vi "solution.vi"() -> ()   [LabVIEW 2015]
doc: "Use this template to build a producer/consumer design pattern with events to produce queue items. Use this design pattern instead of the User Interface Event Handler pattern for user interfaces when you want to execute code asynchronously in response to an event without slowing the user interface responsiveness."
uses:
  Controls/order&data.ctl
  Controls/#status.ctl
  Users Data.ctl
  Controls/User data.ctl
  Controls/Buttons.ctl
  Controls/#status message.ctl
panel:
  in  "error in":errorcluster
  out "error out":errorcluster
  in  "Enter":bool
  in  "User Input":string
  in  "Right Buttons":T1
  out "Right Menu":T2
  in  "Left Buttons":T1
  out "Left Menu":T2
  in  "Card Simulator":bool
  out "ATM Messages":string
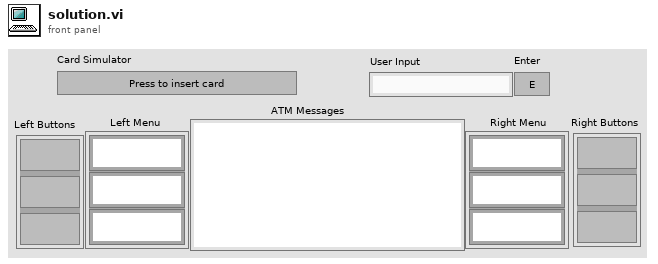
[diagram p1: front panel]
types:
  T1 = cluster{"Func Button":bool, "Func Button 2":bool, "Func Button 3":bool}
  T2 = cluster{"RFS String":string, "RFS String 2":string, "RFS String 3":string}
  T3 = typedef "Buttons.ctl" = cluster{"Left Buttons":cluster{"Func Button":bool, "Func Button 2":bool, "Func Button 3":bool}, "Right Buttons":cluster{"Func Button":bool, "Func Button 2":bool, "Func Button 3":bool}}
  T4 = typedef "Users Data.ctl" = cluster{"Users":T5[], "Customer":T5, "Message":string, "Right Menu":cluster{"RFS String":string, "RFS String 2":string, "RFS String 3":string}, "Left Menu":cluster{"RFS String":string, "RFS String 2":string, "RFS String 3":string}}
  T5 = typedef "User data.ctl" = cluster{"Name":string, "Surname":string, "Cash":i32, "PIN":string}
  T6 = typedef "order&data.ctl" = cluster{"order":T7, "data":string}
  T7 = typedef "#status.ctl" = enum16{"Balance inq", "End of Time", "Show messsage", "Check PIN", "Initialize", "Exit", "Return&Terminate", "Balance Inquiry", "None", "Fast Cash", "Withdraw", "Deposit"}
  T8 = typedef "#status message.ctl" = enum16{"Balance inq", "Withdraw welcome", "Withdraw Failed", "Deposit welcome", "End of Time", "Show messsage", "Check PIN", "Initialize", "Exit", "Return&Terminate", "Balance Inquiry", "None", "First Cash", "Withdraw", "Deposit"}
  T9 = enum8{"Enabled", "Disabled", "Disabled and Grayed Out"}
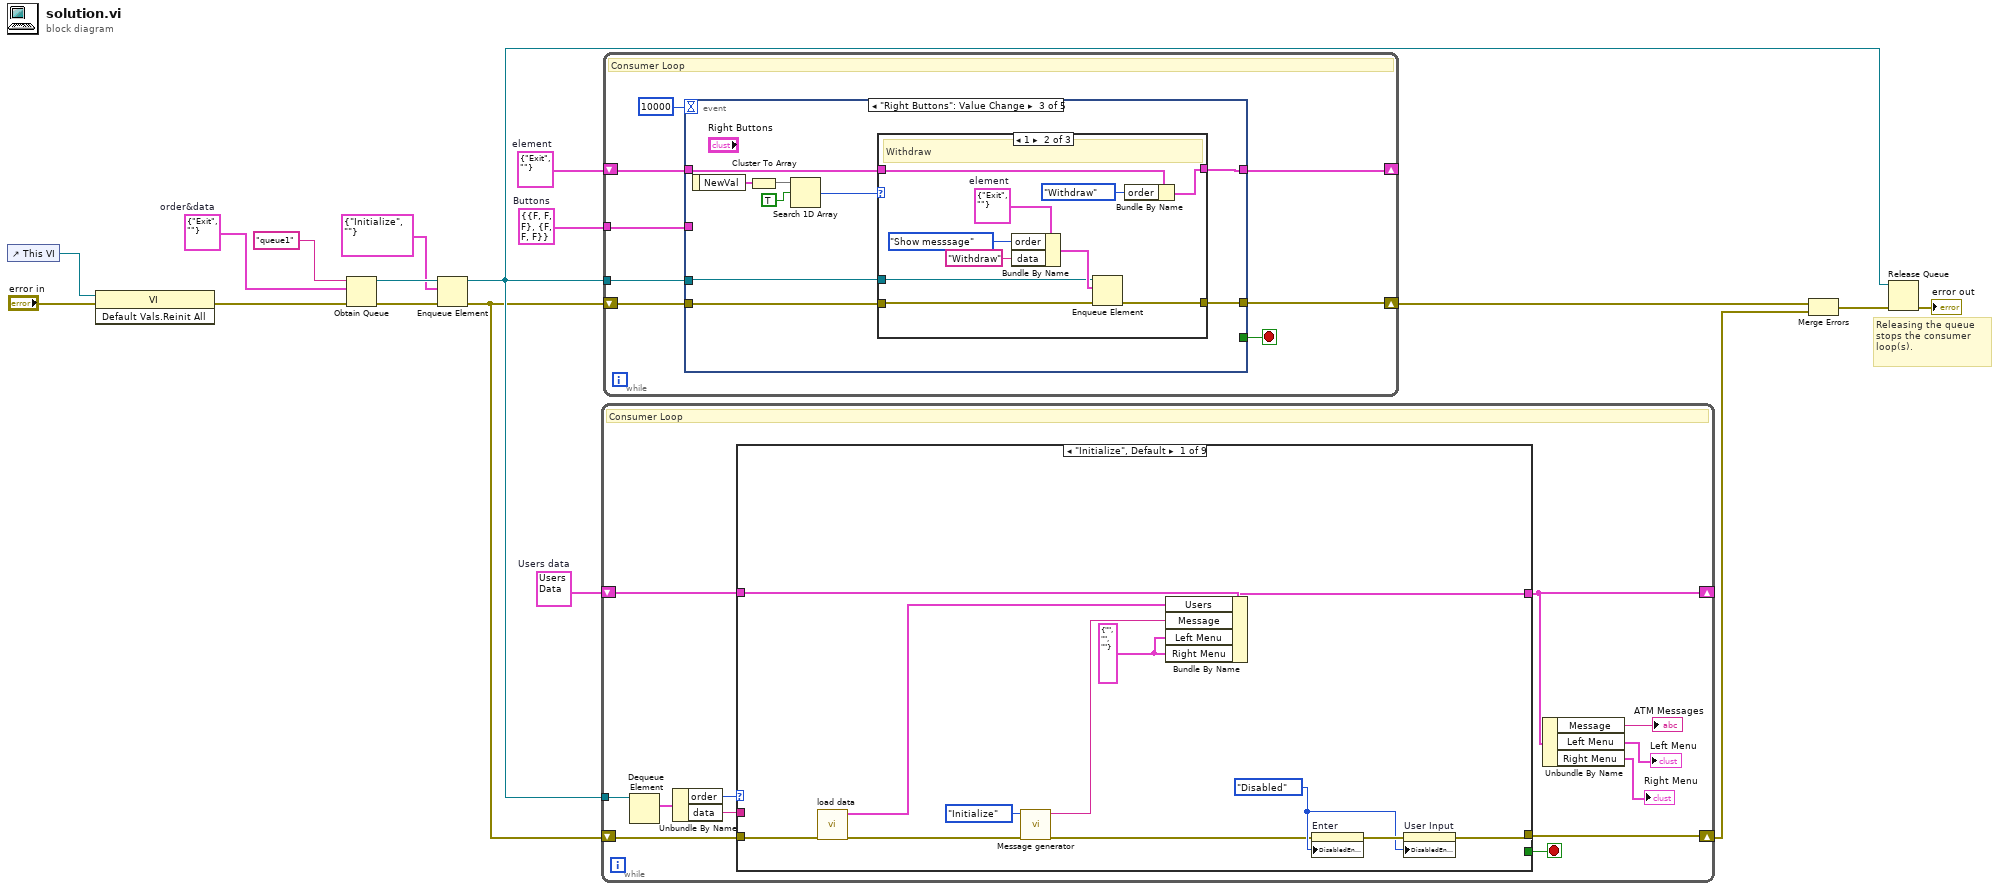
[diagram p0: block diagram]
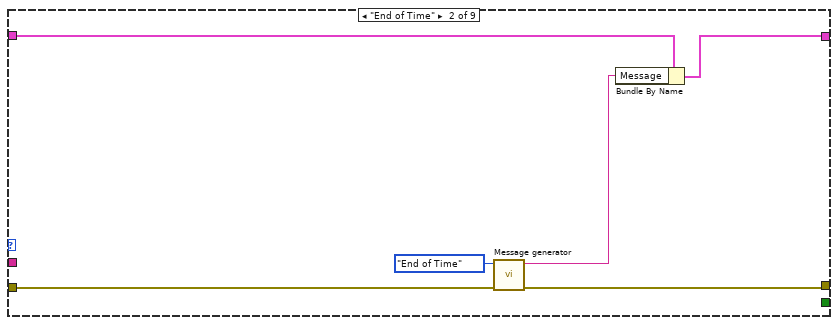
[diagram p2: hidden frame]
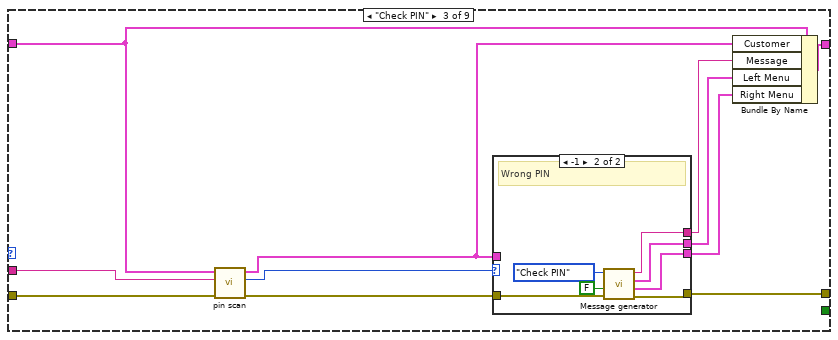
[diagram p3: hidden frame]
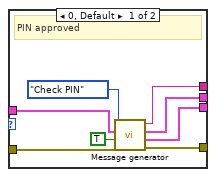
[diagram p4: hidden frame]
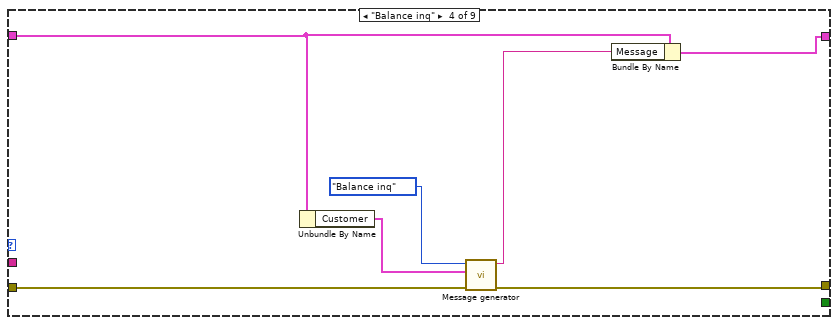
[diagram p5: hidden frame]
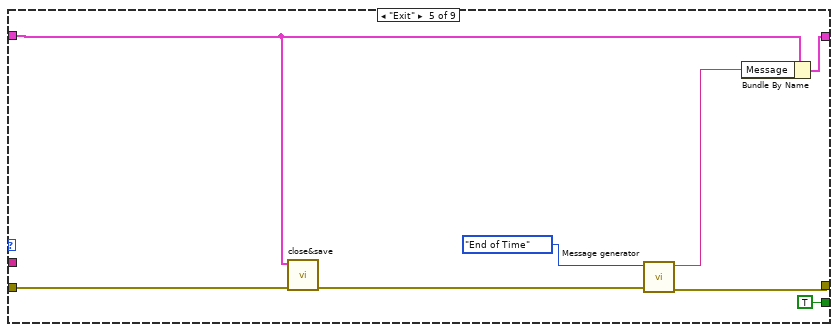
[diagram p6: hidden frame]
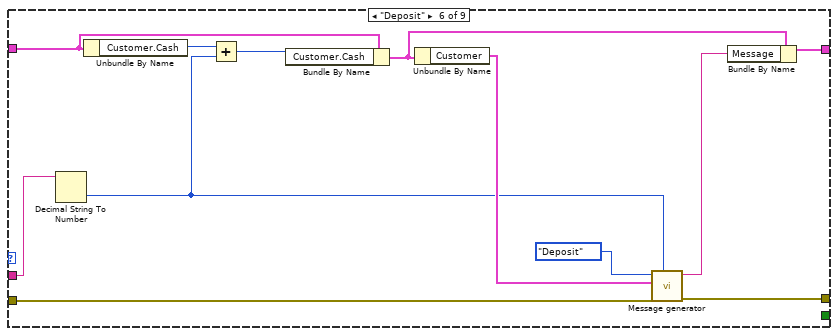
[diagram p7: hidden frame]
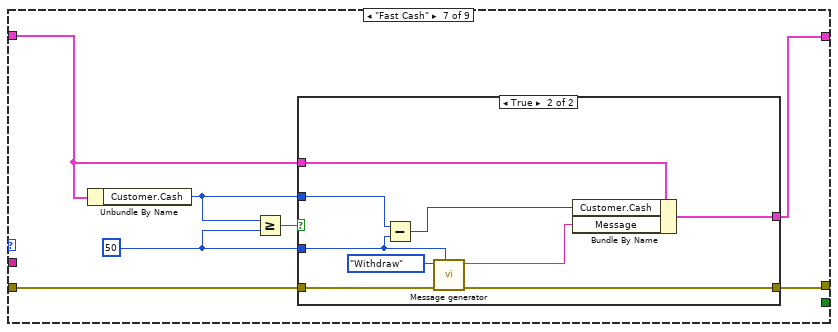
[diagram p8: hidden frame]
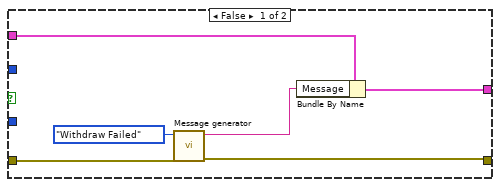
[diagram p9: hidden frame]
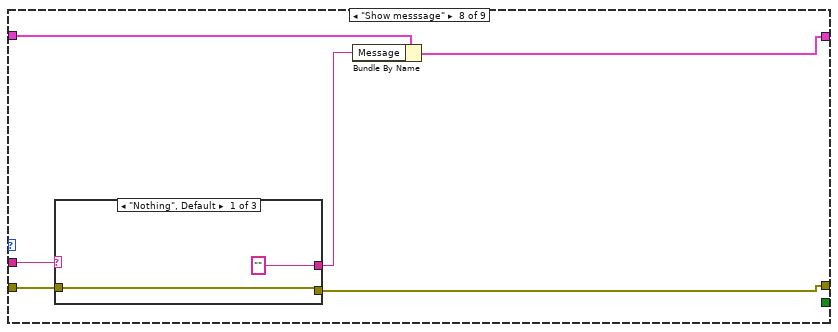
[diagram p10: hidden frame]
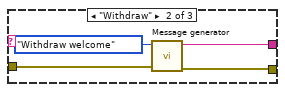
[diagram p11: hidden frame]
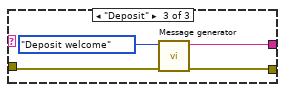
[diagram p12: hidden frame]
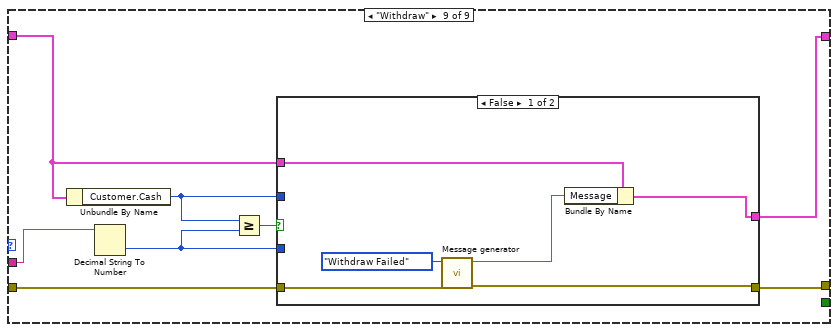
[diagram p13: hidden frame]
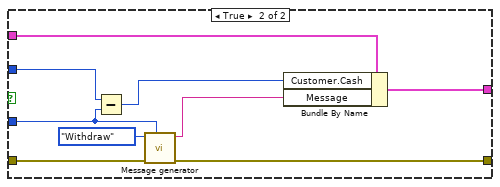
[diagram p14: hidden frame]
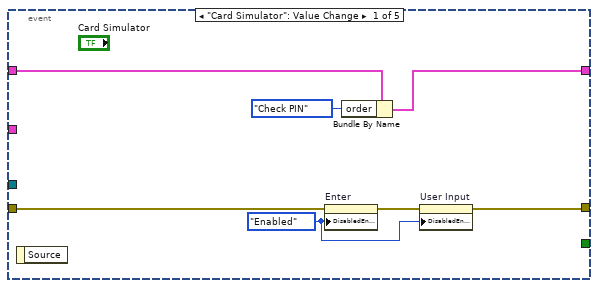
[diagram p15: hidden frame]
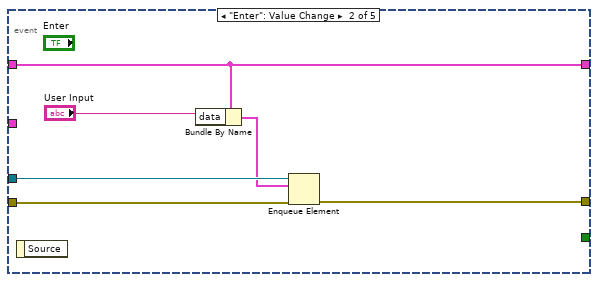
[diagram p16: hidden frame]
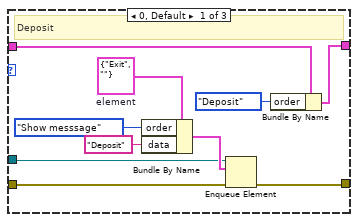
[diagram p17: hidden frame]
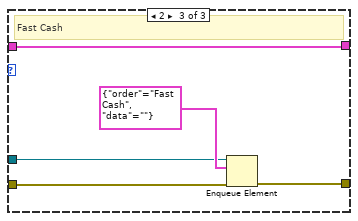
[diagram p18: hidden frame]
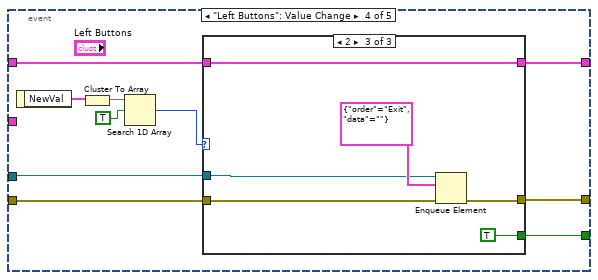
[diagram p19: hidden frame]
diagram:
  w8 = T3 {"Left Buttons"={"Func Button"=FALSE, "Func Button 2"=FALSE, "Func Button 3"=FALSE}, "Right Buttons"={"Func Button"=FALSE, "Func Button 2"=FALSE, "Func Button 3"=FALSE}}  # Buttons
  w9 = T4 {"Users"=[{"Name"="John", "Surname"="Doe", "Cash"=2000, "PIN"=""}, {"Name"="Jennifer", "Surname"="Rodriguez", "Cash"=1500, "PIN"=""}, {"Name"="Bryan", "Surname"="Smith", "Cash"=800, "PIN"=""}, {"Name"="Julie", "Surname"="Ramirez", "Cash"=900, "PIN"=""}], "Customer"={"Name"="", "Surname"="", "Cash"=0, "PIN"=""}, "Message"="", "Right Menu"={"RFS String"="", "RFS String 2"="", "RFS String 3"=""}, "Left Menu"={"RFS String"="", "RFS String 2"="", "RFS String 3"=""}}  # Users data
  w10 = T6 {"order"=enum."Exit", "data"=""}  # element
  w17 = T6 {"order"=enum."Exit", "data"=""}  # order&data
  # "Releasing the queue stops the consumer loop(s)."
  n1 = control-ref of="This VI"() -> (w3:refnum<vi>)
  n2 = invoke class="VI" method="Default Vals.Reinit All"(reference=w3, error in="error in") -> (error out=w2:errorcluster)  [unwired: 1 in, 2 out]
  n3 = Obtain Queue(name (unnamed)="queue1", element data type=w17, error in (no error)=w2) -> (queue out=w14:refnum<queue>, error out=w15:errorcluster)  [unwired: 2 in, 1 out]
  n4 = Enqueue Element(queue=w14, element=T6 {"order"=enum."Initialize", "data"=""} ("order&data 2"), error in (no error)=w15) -> (queue out=w13:refnum<queue>, error out=w11:errorcluster)  [unwired: 1 in, 1 out]
  n5 = while {
    tunnel: w13 -> [w25]
    shift-right: [w22] -> w6
    shift-left: w11 -> [w23]
    shift-right: [w21] -> _
    shift-left: w9 -> [w27]
    stop <- w26 stop-if-true
    # "Consumer Loop"
    n6 = Dequeue Element(queue=w25) -> (element=w29:T6)  [unwired: 2 in, 3 out]
    n7 = Unbundle By Name(w29) -> ("order"=w28:T7, "data"=w24:string)
    n8 = case shown="\"Initialize\", Default" w28 {
      tunnel: w27 -> [w41 w45 w57 w77 w81 w93 w103 w128 w140]
      tunnel: [w39 w44 w55 w75 w87 w95 w102 w127 w139] -> w21
      tunnel: [_ _ _ _ TRUE _ _ _ _] -> w26
      tunnel: w24 -> [_ _ w58 _ _ w100 _ w124 w144]
      tunnel: w23 -> [w34 w47 w49 w80 w83 w97 w105 w126 w146]
      tunnel: [w33 w46 w54 w79 w88 w96 w104 w125 w145] -> w22
      frame "Initialize", Default {
        w31 = T2 {"RFS String"="", "RFS String 2"="", "RFS String 3"=""} ("Left Menu")
        w37 = T9."Disabled" ("Disabled")
        n9 = call "load data.vi"("error in"=w34) -> ("error out"=w36:errorcluster, "Array"=w40:T5[])  [unwired: 9 in]
        n10 = call "Message generator.vi"("error in"=w36, "order"=#status_message."Initialize") -> ("error out"=w35:errorcluster, "message"=w32:string)  [unwired: 6 in, 2 out]
        n11 = Bundle By Name(cluster=w41, "Users"=w40, "Message"=w32, "Left Menu"=w31, "Right Menu"=w31) -> (w39:T4)
        n12 = property on="Enter" class="Bool"(error in=w35, "DisabledEnum"=w37) -> (error out=w38:errorcluster)  [unwired: 1 in, 1 out]
        n13 = property on="User Input" class="Str"(error in=w38, "DisabledEnum"=w37) -> (error out=w33:errorcluster)  [unwired: 1 in, 1 out]
      }
      frame "End of Time" {
        n14 = call "Message generator.vi"("error in"=w47, "order"=#status_message."End of Time") -> ("error out"=w46:errorcluster, "message"=w43:string)  [unwired: 6 in, 2 out]
        n15 = Bundle By Name(cluster=w45, "Message"=w43) -> (w44:T4)
      }
      frame "Check PIN" {
        n16 = call "pin scan.vi"("error in"=w49, "data"=w58, "Users data"=w57) -> ("error out"=w48:errorcluster, "index of element"=w56:i32, "User data"=w53:T5)  [unwired: 6 in]
        n17 = case shown="-1" w56 {
          tunnel: [w64 w72] -> w52
          tunnel: w48 -> [w66 w71]
          tunnel: [w65 w70] -> w54
          tunnel: w53 -> [w62 _]
          tunnel: [w61 w69] -> w51
          tunnel: [w60 w68] -> w50
          frame 0, Default {
            # "PIN approved"
            n18 = call "Message generator.vi"("error in"=w66, "correct pin"=TRUE, "Customer"=w62, "order"=#status_message."Check PIN") -> ("error out"=w65:errorcluster, "Right Menu"=w60:T2, "Left Menu"=w61:T2, "message"=w64:string)  [unwired: 4 in]
          }
          frame -1 {
            # "Wrong PIN"
            n19 = call "Message generator.vi"("error in"=w71, "correct pin"=FALSE, "order"=#status_message."Check PIN") -> ("error out"=w70:errorcluster, "Right Menu"=w68:T2, "Left Menu"=w69:T2, "message"=w72:string)  [unwired: 5 in]
          }
        }
        n20 = Bundle By Name(cluster=w57, "Customer"=w53, "Message"=w52, "Left Menu"=w51, "Right Menu"=w50) -> (w55:T4)
      }
      frame "Balance inq" {
        n21 = Unbundle By Name(w77) -> ("Customer"=w78:T5)
        n22 = call "Message generator.vi"("error in"=w80, "Customer"=w78, "order"=#status_message."Balance inq") -> ("error out"=w79:errorcluster, "message"=w76:string)  [unwired: 5 in, 2 out]
        n23 = Bundle By Name(cluster=w77, "Message"=w76) -> (w75:T4)
      }
      frame "Exit" {
        n24 = call "close&save.vi"("error in"=w83, "input cluster"=w81) -> ("error out"=w82:errorcluster)  [unwired: 9 in]
        n25 = call "Message generator.vi"("error in"=w82, "order"=#status_message."End of Time") -> ("error out"=w88:errorcluster, "message"=w86:string)  [unwired: 6 in, 2 out]
        n26 = Bundle By Name(cluster=w81, "Message"=w86) -> (w87:T4)
      }
      frame "Deposit" {
        n27 = Decimal String To Number(string=w100) -> (number=w89:i32)  [unwired: 2 in, 1 out]
        n28 = Unbundle By Name(w93) -> ("Customer.Cash"=w99:i32)
        n29 = Add(x=w99, y=w89) -> (x+y=w98:i32)
        n30 = Bundle By Name(cluster=w93, "Customer.Cash"=w98) -> (w92:T4)
        n31 = Unbundle By Name(w92) -> ("Customer"=w91:T5)
        n32 = call "Message generator.vi"("cash"=w89, "error in"=w97, "Customer"=w91, "order"=#status_message."Deposit") -> ("error out"=w96:errorcluster, "message"=w94:string)  [unwired: 4 in, 2 out]
        n33 = Bundle By Name(cluster=w92, "Message"=w94) -> (w95:T4)
      }
      frame "Fast Cash" {
        w101 = 50 ("y")
        n34 = Unbundle By Name(w103) -> ("Customer.Cash"=w106:i32)
        n35 = Greater Or Equal?(x=w106, y=w101) -> (x >= y?=w107:bool)
        n36 = case shown="True" w107 {
          tunnel: w105 -> [w113 w122]
          tunnel: [w112 w121] -> w104
          tunnel: w101 -> [_ w115]
          tunnel: w106 -> [_ w120]
          tunnel: w103 -> [w111 w119]
          tunnel: [w108 w114] -> w102
          frame False {
            n37 = call "Message generator.vi"("error in"=w113, "order"=#status_message."Withdraw Failed") -> ("error out"=w112:errorcluster, "message"=w109:string)  [unwired: 6 in, 2 out]
            n38 = Bundle By Name(cluster=w111, "Message"=w109) -> (w108:T4)
          }
          frame True {
            n39 = Subtract(x=w120, y=w115) -> (x-y=w118:i32)
            n40 = call "Message generator.vi"("cash"=w115, "error in"=w122, "order"=#status_message."Withdraw") -> ("error out"=w121:errorcluster, "message"=w117:string)  [unwired: 5 in, 2 out]
            n41 = Bundle By Name(cluster=w119, "Customer.Cash"=w118, "Message"=w117) -> (w114:T4)
          }
        }
      }
      frame "Show messsage" {
        n42 = case shown="\"Nothing\", Default" w124 {
          tunnel: w126 -> [w130 w134 w138]
          tunnel: [w130 w133 w137] -> w125
          tunnel: ["" ("message") w132 w136] -> w123
          frame "Nothing", Default {
          }
          frame "Withdraw" {
            n43 = call "Message generator.vi"("error in"=w134, "order"=#status_message."Withdraw welcome") -> ("error out"=w133:errorcluster, "message"=w132:string)  [unwired: 6 in, 2 out]
          }
          frame "Deposit" {
            n44 = call "Message generator.vi"("error in"=w138, "order"=#status_message."Deposit welcome") -> ("error out"=w137:errorcluster, "message"=w136:string)  [unwired: 6 in, 2 out]
          }
        }
        n45 = Bundle By Name(cluster=w128, "Message"=w123) -> (w127:T4)
      }
      frame "Withdraw" {
        n46 = Unbundle By Name(w140) -> ("Customer.Cash"=w141:i32)
        n47 = Decimal String To Number(string=w144) -> (number=w142:i32)  [unwired: 2 in, 1 out]
        n48 = Greater Or Equal?(x=w141, y=w142) -> (x >= y?=w143:bool)
        n49 = case shown="False" w143 {
          tunnel: w146 -> [w152 w161]
          tunnel: [w151 w160] -> w145
          tunnel: w142 -> [_ w154]
          tunnel: w141 -> [_ w159]
          tunnel: w140 -> [w150 w158]
          tunnel: [w147 w153] -> w139
          frame False {
            n50 = call "Message generator.vi"("error in"=w152, "order"=#status_message."Withdraw Failed") -> ("error out"=w151:errorcluster, "message"=w148:string)  [unwired: 6 in, 2 out]
            n51 = Bundle By Name(cluster=w150, "Message"=w148) -> (w147:T4)
          }
          frame True {
            n52 = Subtract(x=w159, y=w154) -> (x-y=w157:i32)
            n53 = call "Message generator.vi"("cash"=w154, "error in"=w161, "order"=#status_message."Withdraw") -> ("error out"=w160:errorcluster, "message"=w156:string)  [unwired: 5 in, 2 out]
            n54 = Bundle By Name(cluster=w158, "Customer.Cash"=w157, "Message"=w156) -> (w153:T4)
          }
        }
      }
    }
    n55 = Unbundle By Name(w21) -> ("Message"=→"ATM Messages":string, "Left Menu"=→"Left Menu":T2, "Right Menu"=→"Right Menu":T2)
  }
  n56 = while {
    shift-right: [w167] -> w7
    shift-left: w11 -> [w168]
    tunnel: w13 -> [w169]
    shift-right: [w165] -> _
    shift-left: w10 -> [w166]
    tunnel: w8 -> [w162]
    stop <- w163 stop-if-true
    # "Consumer Loop"
    n57 = event shown="[2] \"Right Buttons\": Value Change" {
      selector: _ -> [_ _ _ _ _]
      dyn-events: _ -> [_ _ _ _ _]
      timeout: 10000 -> [_ _ _ _ _]
      tunnel: w169 -> [_ w180 w189 w224 w241]
      tunnel: w168 -> [w173 w182 w191 w226 w243]
      tunnel: [w171 w181 w190 w225 w242] -> w167
      tunnel: w166 -> [w176 w179 w184 w223 _]
      tunnel: [w175 w179 w183 w222 _] -> w165
      tunnel: [_ _ _ w217 _] -> w163
      tunnel: w162 -> [_ _ _ _ _]
      event "Card Simulator": Value Change {
        w170 = T9."Enabled" ("Disabled")
        n58 = event-data() -> ()  [unwired: 1 in, 1 out]
        n59 = property on="Enter" class="Bool"(error in=w173, "DisabledEnum"=w170) -> (error out=w172:errorcluster)  [unwired: 1 in, 1 out]
        n60 = Bundle By Name(cluster=w176, "order"=#status."Check PIN") -> (w175:T6)
        n61 = property on="User Input" class="Str"(error in=w172, "DisabledEnum"=w170) -> (error out=w171:errorcluster)  [unwired: 1 in, 1 out]
      }
      event "Enter": Value Change {
        n62 = event-data() -> ()  [unwired: 1 in, 1 out]
        n63 = Bundle By Name(cluster=w179, "data"="User Input") -> (w178:T6)
        n64 = Enqueue Element(queue=w180, element=w178, error in (no error)=w182) -> (error out=w181:errorcluster)  [unwired: 1 in, 2 out]
      }
      event "Right Buttons": Value Change {
        n65 = event-data() -> ("NewVal"=w188:T1)  [unwired: 1 in]
        n66 = Cluster To Array(cluster=w188) -> (array=w187:bool[])
        n67 = Search 1D Array(1D array=w187, element=TRUE) -> (index of element=w185:i32)  [unwired: 1 in]
        n68 = case shown="1" w185 {
          tunnel: w191 -> [w196 w206 w215]
          tunnel: [w195 w205 w214] -> w190
          tunnel: w189 -> [w192 w202 w212]
          tunnel: w184 -> [w194 w204 w213]
          tunnel: [w193 w203 w213] -> w183
          frame 0, Default {
            w198 = T6 {"order"=enum."Exit", "data"=""}  # element
            # "Deposit"
            n69 = Bundle By Name(cluster=w198, "order"=#status."Show messsage", "data"="Deposit") -> (w200:T6)
            n70 = Enqueue Element(queue=w192, element=w200, error in (no error)=w196) -> (error out=w195:errorcluster)  [unwired: 1 in, 2 out]
            n71 = Bundle By Name(cluster=w194, "order"=#status."Deposit") -> (w193:T6)
          }
          frame 1 {
            w210 = T6 {"order"=enum."Exit", "data"=""}  # element
            # "Withdraw"
            n72 = Bundle By Name(cluster=w210, "order"=#status."Show messsage", "data"="Withdraw") -> (w208:T6)
            n73 = Enqueue Element(queue=w202, element=w208, error in (no error)=w206) -> (error out=w205:errorcluster)  [unwired: 1 in, 2 out]
            n74 = Bundle By Name(cluster=w204, "order"=#status."Withdraw") -> (w203:T6)
          }
          frame 2 {
            # "Fast Cash"
            n75 = Enqueue Element(queue=w212, element=T6 {"order"=enum."Fast Cash", "data"=""}, error in (no error)=w215) -> (error out=w214:errorcluster)  [unwired: 1 in, 2 out]
          }
        }
      }
      event "Left Buttons": Value Change {
        n76 = event-data() -> ("NewVal"=w219:T1)  [unwired: 1 in]
        n77 = Cluster To Array(cluster=w219) -> (array=w221:bool[])
        n78 = Search 1D Array(1D array=w221, element=TRUE) -> (index of element=w218:i32)  [unwired: 1 in]
        n79 = case shown="2" w218 {
          tunnel: w226 -> [w228 w233 w238]
          tunnel: [w228 w232 w237] -> w225
          tunnel: w224 -> [_ w231 w236]
          tunnel: w223 -> [w227 w229 w234]
          tunnel: [w227 w229 w234] -> w222
          tunnel: [_ _ TRUE] -> w217
          frame 0, Default {
          }
          frame 1 {
            n80 = Enqueue Element(queue=w231, element=T6 {"order"=enum."Balance inq", "data"=""}, error in (no error)=w233) -> (error out=w232:errorcluster)  [unwired: 1 in, 2 out]
          }
          frame 2 {
            n81 = Enqueue Element(queue=w236, element=T6 {"order"=enum."Exit", "data"=""}, error in (no error)=w238) -> (error out=w237:errorcluster)  [unwired: 1 in, 2 out]
          }
        }
      }
      event Timeout {
        n82 = event-data() -> ()  [unwired: 1 in, 1 out]
        n83 = Enqueue Element(queue=w241, element=T6 {"order"=enum."End of Time", "data"=""}, error in (no error)=w243) -> (error out=w242:errorcluster)  [unwired: 1 in, 2 out]
      }
    }
  }
  n84 = Merge Errors(w7, w6) -> (w5:errorcluster)
  n85 = Release Queue(queue=w13, error in (no error)=w5) -> (error out=→"error out":errorcluster)  [unwired: 1 in, 2 out]
